vi "Version4.0.vi"() -> ()   [LabVIEW 2012]
uses:
  <vilib>/Instr/_visa.llb/VISA Configure Serial Port (Instr).vi
  Function_Set/Debug/Function_Set.dll
panel:
  in  "选项卡控件":T1(tab)
  in  "查询 2":bool
  in  "Other:":string
  in  "Save This Shot":bool
  out "Shots:":i32
  in  "Save This Notes":bool
  in  "Other Notes:":string
  out "Shot's situation:":string
  out "Shots:":i32
  out "Notes:":string
  in  "查询":bool
  in  "Options":u16(ring) caption="Choose File:" items=["2014-5-27梁一寒-Notes.txt", "2014-5-27梁一寒.txt", "2014-5-27袁鹏-Notes.txt", "2014-5-27袁鹏.txt", "20140527_110114.txt", "20140527_110114combined.txt", "20140527_110235.txt", "20140527_110235combined.txt"]
  in  "Initial Folder Path:":path
  in  "透镜位置：":dbl
  in  "靶位置：":dbl
  in  "激光能量：":dbl
  in  "实验员":u16(ring)
  in  "查找实验员":u16(ring)
  in  "搜索结果":u16(ring) caption="查找结果:" items=["2014-5-27梁一寒-Notes.txt", "2014-5-27梁一寒.txt"]
  in  "?":bool
  in  "Your Own:":u16(ring) items=["2, 0, 3, 2"]
  in  "FrameStartTriggerMode":T2(ring)
  in  "AcquisitionMode":T3(ring)
  in  "ExposureMode":T4(ring)
  in  "AVT SDK Demon":bool
  out "CCD ID":string
  out "ExposureMode":string
  out "ExposureValue":u32
  out "AcquisitionMode":string
  out "FrameStartTriggerMode":string
  in  "ExposureValue":u32
  in  "CameraStart":bool
  in  "CameraStop":bool
  in  "CameraSet":bool
  in  "CameraGet":bool
  in  "CameraSetAll":bool
  in  "path to JPEG file":path caption="Path of the Pic"
  out "new picture":picture caption="Pic"
  in  "OPEN":bool
  in  "端口选择":refnum<visa-resource-name>="COM1"
  in  "baud rate":u32=9600
  in  "data bits":u16=8
  in  "stop bits":u16(ring)=10 items=["1.0"=10, "1.5"=15, "2.0"=20]
  in  "flow control":u16(ring) items=["None"=0, "XON/XOFF"=1, "RTS/CTS"=2, "DTR/DSR"=4]
  in  "timeout":u32=10
  in  "RS485地址":string="12"
  in  "读取间隔(s)":dbl=1.0 caption="Delay Time (s)"
  in  "数据文件夹":string="data"
  in  "记录说明":string="test"
  out "数据路径":path
  in  "parity (0:none)":enum16{"None", "Odd", "Even", "Mark", "Space"}(ring)
  in  "记录所有读取数据?":bool
  out "已记录数据点":u32 caption="recorded number"
  in  "stop":bool
  out "电离规图表":dbl(graph)
  out "电阻规图表":dbl(graph)
  out "已读取数据点":i32
  out "预定耗时":dbl
  out "实际耗时":dbl
  in  "临界压强(Pa)":dbl=8.0
  in  "圈数":i32
  in  "X边长（mm）":dbl
  in  "VISA resource name":refnum<visa-resource-name>="COM1"
  in  "确认":bool
  in  "X轴速度mm/s":dbl(knob) scale=0.0..100.0
  in  "Y边长（mm）":dbl
  in  "Y轴速度mm/s":dbl(knob) scale=0.0..100.0
  out "进度条":dbl(slide) scale=0.0..100.0
  in  "设置速度":bool
  in  "baud rate 2":u32=9600
  in  "VISA resource name 2":refnum<visa-resource-name>="COM1"
  in  "data bits 2":u16=8 min=5 max=8 step=1
  in  "parity":u16(ring) items=["None", "Odd", "Even", "Mark", "Space"]
  in  "stop bits 2":u16(ring)=10 items=["1.0"=10, "1.5"=15, "2.0"=20]
  in  "timeout (ms)":u32=10000
  in  "flow control 2":u16(ring) items=["None"=0, "XON/XOFF"=1, "RTS/CTS"=2, "DTR/DSR"=4]
  in  "Input\nbuffer size":u32=4096
  in  "激光器端口设置完毕":bool
  in  "读取激光器字符串":string
  in  "控制器端口设置完毕":bool
  in  "baud rate 3":u32=9600
  in  "VISA resource name 3":refnum<visa-resource-name>="COM1"
  in  "data bits 3":u16=8 min=5 max=8 step=1
  in  "parity 2":u16(ring) items=["None", "Odd", "Even", "Mark", "Space"]
  in  "stop bits 3":u16(ring)=10 items=["1.0"=10, "1.5"=15, "2.0"=20]
  in  "timeout (ms) 2":u32=10000
  in  "flow control 3":u16(ring) items=["None"=0, "XON/XOFF"=1, "RTS/CTS"=2, "DTR/DSR"=4]
  in  "Input buffer size 2":u32=4096
  in  "字符串输出":bool
  in  "直接使用字符串输入：":string
  in  "启动总开关":bool
  in  "All the commands":path
  in  "选项卡控件 2":enum32{"单轴控制", "四轴控制", "同步控制"}(tab)
  in  "单轴输入":bool
  in  "Number of Pulses":i16
  in  "模式转换":bool
  in  "回到机械原点":bool
  in  "选择轴":u16(ring)=1 items=["轴1"=1, "轴2"=2, "轴3"=3, "轴4"=4]
  in  "轴 4":i16
  in  "轴 5":i16
  in  "轴 6":i16
  in  "轴1 2":i16
  in  "模式转换 2":bool
  in  "多轴输入":bool
  in  "模式转换 3":bool
  in  "轴1":i16
  in  "轴2":i16
  in  "轴3":i16
  in  "轴4":i16
  in  "同步运作":bool
  out "正在移动":bool
  in  "询问状态":bool
  in  "Parameter":string
  in  "轴":u16(ring)=1 items=["未定义", "轴1", "轴2", "轴3", "轴4"]
  out "情况":string
  in  "速度设置":bool
  in  "加速时间（ms）":i32
  in  "最大速度（PPS）":i32
  in  "最小速度（PPS）":i32
  in  "轴 3":u16(ring)=1 items=["未定义", "轴1", "轴2", "轴3", "轴4"]
  in  "返回位置":bool
  out "位置返回值":string
  in  "步长设置":bool
  in  "轴 2":u16(ring)=1 items=["未定义", "轴1", "轴2", "轴3", "轴4"]
  in  "分割步长":u16(ring) items=["0.36°;1000p/c;1μm"=2, "0.18°;2000p/c;0.5μm"=4, "0.036°;10000p/c;0.1μm"=20, "0.018°;20000p/c;0.05μm"=40, "0.0036°;100000p/c;0.01μm"=200]
  in  "全部减速停止":bool
  in  "轴4减速停止":bool
  in  "轴3减速停止":bool
  in  "轴2减速停止":bool
  in  "轴1减速停止":bool
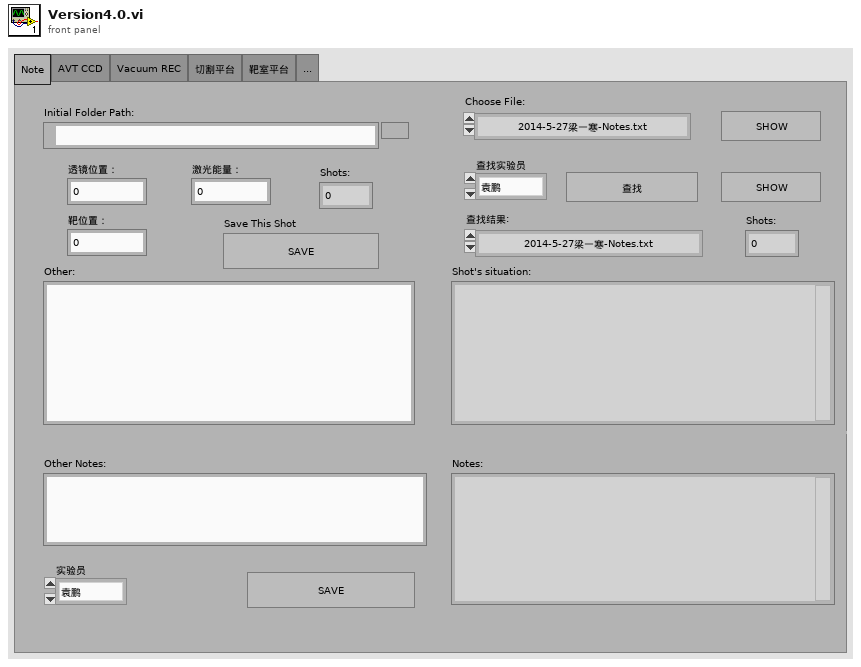
[diagram p1: front panel]
types:
  T1 = enum32{"Note", "AVT CCD", "Vacuum REC", "切割平台", "靶室平台", "..."}
  T2 = enum16{"默认", "Freerun", "SyncIn1", "SyncIn2", "FixedRate", "Software"}
  T3 = enum16{"默认", "Continuous", "SingleFrame", "MultiFrame", "Recorder"}
  T4 = enum16{"默认", "Manual", "Auto", "AutoOnce", "External"}
  T5 = enum16{"open", "replace", "create", "open or create", "replace or create", "replace or create with confirmation"}
  T6 = typedef "imagedata.ctl" = cluster{"image type":i32, "image depth":i32, "image":u8[], "mask":u8[], "colors":u32[], "Rectangle":cluster{"left":i16, "top":i16, "right":i16, "bottom":i16}}
  T7 = cluster{"Resister":dbl, "Ionization":dbl, "time":string, "Ionization":dbl, "Ionization":dbl, u32, i32}
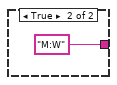
[diagram p4: hidden frame]
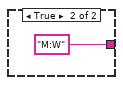
[diagram p11: hidden frame]
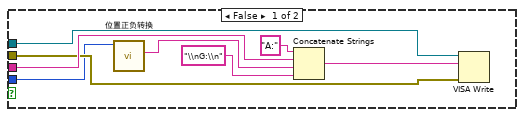
[diagram p13: hidden frame]
diagram:
  n1 = while {
    tunnel: "选项卡控件" -> [w19]
    stop <- w20 continue-if-true
    n2 = property on="Options" class="Ring (严格)"() -> ("Strings []"=w15:string[])  [unwired: 2 in, 2 out]
    n3 = property on="查找实验员" class="Ring (严格)"() -> ("RingText.Text"=w16:string)  [unwired: 2 in, 2 out]
    n4 = property on="实验员" class="Ring (严格)"() -> ("RingText.Text"=w17:string)  [unwired: 2 in, 2 out]
    n5 = property on="搜索结果" class="Ring (严格)"() -> ("RingText.Text"=w4:string)  [unwired: 2 in, 2 out]
    n6 = Array Size(array=w15) -> (size(s)=w14:i32)
    n7 = Equal?(x=T1."Note", y=w19) -> (x = y?=w20:bool)
    n8 = Not Equal?(x="查询", y="查询 2") -> (x != y?=w3:bool)
    n9 = Equal?(x="查询", y=w3) -> (x = y?=w8:bool)
    n10 = case shown="真" "Save This Shot" {
      tunnel: "Initial Folder Path:" -> [_ w97]
      tunnel: w17 -> [_ w85]
      frame False {
      }
      frame True {
        n11 = property on="Shots:" class="DigNum (严格)"() -> ("Value"=w93:i32)  [unwired: 2 in, 2 out]
        n12 = Decrement(x=w93) -> (x-1=w92:i32)
        n13 = Get Date/Time String(date format (0)=enum16{"short", "long", "abbreviated"}."short" ("日期格式(0)")) -> (date string=w108:string)  [unwired: 2 in, 1 out]
        n14 = feedback #1(1.0 ("x")) -> (w100:dbl)
        n15 = Increment(x=w100) -> (x+1=w98:dbl)
        "Shots:" <- w98
        n16 = feedback-in #1(w98) -> ()
        n17 = Search and Replace String(replace all?=TRUE ("替换全部？(F)"), input string=w108, search string="/" ("搜索字符串"), replace string="-" ("替换字符串(\"\")")) -> (result string=w105:string)  [unwired: 4 in, 3 out]
        n18 = Concatenate Strings(w105, "-" ("字符串"), w85, ".txt" ("字符串")) -> (w109:string)
        n19 = Build Path(base path=w97, name or relative path=w109) -> (appended path=w110:path)
        n20 = Open/Create/Replace File(file path (use dialog)=w110, operation (0:open)=T5."open or create" ("操作(0:open)"), access (0:read/write)=enum16{"read/write", "read-only", "write-only"}."read/write" ("权限(0:read/write)")) -> (refnum out=w102:refnum<file>)  [unwired: 3 in, 2 out]
        n21 = Number To Decimal String(number=w92) -> (decimal integer string=w96:string)  [unwired: 1 in]
        n22 = Concatenate Strings("NO." ("字符串"), w96, ": ;透镜位置: %f ;靶位置: %f ;激光能量: %f ;Other: %s\\n" ("格式字符串")) -> (w90:string)
        n23 = Set File Position(refnum=w102, from (0:start)=enum16{"start", "end", "current"}."end" ("自（0:起始）")) -> (refnum out=w101:refnum<file>)  [unwired: 2 in, 1 out]
        n24 = Format Into String(format string=w90, initial string=w101, "透镜位置：", "靶位置：", "激光能量：", "Other:") -> ()  [unwired: 1 in, 2 out]
      }
    }
    n25 = List Folder(path="Initial Folder Path:") -> (path out=w7:path, filenames=w11:string[])  [unwired: 3 in, 2 out]
    n26 = case shown="真" "Save This Notes" {
      tunnel: "Initial Folder Path:" -> [_ w68]
      tunnel: w17 -> [_ w66]
      frame False {
      }
      frame True {
        n27 = Get Date/Time String(date format (0)=enum16{"short", "long", "abbreviated"}."short" ("日期格式(0)")) -> (date string=w79:string)  [unwired: 2 in, 1 out]
        n28 = Search and Replace String(replace all?=TRUE ("替换全部？(F)"), input string=w79, search string="/" ("搜索字符串"), replace string="-" ("替换字符串(\"\")")) -> (result string=w70:string)  [unwired: 4 in, 3 out]
        n29 = Concatenate Strings(w70, "-" ("字符串"), w66, "-Notes.txt" ("字符串")) -> (w69:string)
        n30 = Build Path(base path=w68, name or relative path=w69) -> (appended path=w80:path)
        n31 = Open/Create/Replace File(file path (use dialog)=w80, operation (0:open)=T5."open or create" ("操作(0:open)"), access (0:read/write)=enum16{"read/write", "read-only", "write-only"}."read/write" ("权限(0:read/write)")) -> (refnum out=w73:refnum<file>)  [unwired: 3 in, 2 out]
        n32 = Set File Position(refnum=w73, from (0:start)=enum16{"start", "end", "current"}."end" ("自（0:起始）")) -> (refnum out=w72:refnum<file>)  [unwired: 2 in, 1 out]
        n33 = Format Into String(format string="Other Notes: %s\\n\\n" ("格式字符串"), initial string=w72, "Other Notes:") -> ()  [unwired: 1 in, 2 out]
      }
    }
    n34 = case shown="真" "?" {
      tunnel: w16 -> [_ w31]
      tunnel: w15 -> [_ w30]
      tunnel: w14 -> [_ w29]
      frame False {
      }
      frame True {
        n35 = while {
          tunnel: w30 -> [w38]
          tunnel: w31 -> [w37]
          tunnel: w29 -> [w36]
          i -> [w34]
          stop <- w35 stop-if-true
          n36 = Equal?(x=w36, y=w34) -> (x = y?=w35:bool)
          n37 = Decrement(x=w34) -> (x-1=w33:i32)
          n38 = Index Array(array=w38, index=w33) -> (element=w32:string)
          n39 = Search and Replace String(input string=w32, search string=w37) -> (number of replacements=w39:i32)  [unwired: 6 in, 3 out]
          n40 = Not Equal To 0?(x=w39) -> (x != 0?=w40:bool)
          n41 = case shown="真" w40 {
            tunnel: w32 -> [_ w43]
            frame False {
            }
            frame True {
              n42 = feedback #2() -> (w42:string[])  [unwired: 1 in]
              n43 = Build Array (concatenate)(w42, w43) -> (w41:string[])
              n44 = feedback-in #2(w41) -> ()
              n45 = property on="搜索结果" class="Ring (严格)"("Strings []"=w41) -> ()  [unwired: 2 in, 2 out]
            }
          }
        }
      }
    }
    n46 = property on="Options" class="Ring (严格)"("Strings []"=w11) -> ()  [unwired: 2 in, 2 out]
    n47 = Index Array(array=w11, index="Options") -> (element=w6:string)
    n48 = case shown="真" w8 {
      tunnel: w7 -> [w25 w28]
      tunnel: w6 -> [_ w27]
      tunnel: [w23 w26] -> w5
      tunnel: w4 -> [w24 _]
      frame False {
        n49 = Build Path(base path=w25, name or relative path=w24) -> (appended path=w23:path)
      }
      frame True {
        n50 = Build Path(base path=w28, name or relative path=w27) -> (appended path=w26:path)
      }
    }
    n51 = case shown="真" w3 {
      tunnel: w5 -> [_ w45]
      frame False {
      }
      frame True {
        n52 = Path To String(path=w45) -> (string=w44:string)
        n53 = call "时间延迟2"() -> ()  [unwired: 11 in, 1 out]
        n54 = Search and Replace String(input string=w44, search string="Notes" ("搜索字符串")) -> (number of replacements=w47:i32)  [unwired: 6 in, 3 out]
        n55 = Not Equal To 0?(x=w47) -> (x != 0?=w46:bool)
        n56 = case shown="真" w46 {
          tunnel: w45 -> [w49 w63]
          frame False {
            n57 = Open/Create/Replace File(file path (use dialog)=w49, operation (0:open)=T5."open" ("操作(0:open)"), access (0:read/write)=enum16{"read/write", "read-only", "write-only"}."read-only" ("权限(0:read/write)")) -> (refnum out=w60:refnum<file>)  [unwired: 3 in, 2 out]
            n58 = Read from Text File(file (use dialog)=w60) -> (text=w56:string)  [unwired: 3 in, 3 out]
            n59 = Search and Replace String(replace all?=TRUE ("替换全部？(F)"), input string=w56, search string="\n" ("搜索字符串"), replace string="\n\n" ("替换字符串(\"\")")) -> (result string=w53:string, number of replacements=→"Shots:":i32)  [unwired: 4 in, 2 out]
            n60 = Search and Replace String(replace all?=TRUE ("替换全部？(F)"), input string=w53, search string=";" ("搜索字符串"), replace string="\n" ("替换字符串(\"\")")) -> (result string=→"Shot's situation:":string)  [unwired: 4 in, 3 out]
          }
          frame True {
            n61 = Read from Text File(file (use dialog)=w63) -> (text=→"Notes:":string)  [unwired: 3 in, 3 out]
          }
        }
      }
    }
    n62 = call "时间延迟"() -> ()  [unwired: 11 in, 1 out]
  }
  n63 = while {
    tunnel: "选项卡控件" -> [w117]
    stop <- w118 continue-if-true
    n64 = case shown="真" "OPEN" {
      frame False {
      }
      frame True {
        n65 = call <vilib>:"Read JPEG File.vi"("path to JPEG file"="path to JPEG file") -> ("image data"=w128:T6)  [unwired: 8 in, 2 out]
        n66 = call <vilib>:"Draw Flattened Pixmap.vi"("image data"=w128) -> ("new picture"=→"new picture":picture)  [unwired: 8 in]
      }
    }
    n67 = case shown="真" "CameraStart" {
      frame False {
      }
      frame True {
        n68 = dll-call lib="F:/Kun's Test/Function_Set/Debug/Function_Set.dll" fn="CameraStart"() -> ()  [unwired: 4 in, 2 out]
      }
    }
    n69 = case shown="真" "CameraStop" {
      frame False {
      }
      frame True {
        n70 = dll-call lib="F:/Kun's Test/Function_Set/Debug/Function_Set.dll" fn="CameraStop"() -> ()  [unwired: 4 in, 2 out]
      }
    }
    n71 = case shown="真" "CameraSetAll" {
      frame False {
      }
      frame True {
        n72 = property on="Your Own:" class="Ring (严格)"() -> ("RingText.Text"=w131:string)  [unwired: 2 in, 2 out]
        n73 = Scan From String(format string="%d, %d, %d, %d" ("格式字符串"), input string=w131) -> (output 1=w133:i32, output 2=w134:i32, output 3=w135:i32, output 4=w136:i32)  [unwired: 6 in, 3 out]
        n74 = dll-call lib="F:/Kun's Test/Function_Set/Debug/Function_Set.dll" fn="CameraModeSet"("EM"=w133, "EV"=w134, "AM"=w135, "FSTM"=w136) -> ()  [unwired: 8 in, 2 out]
      }
    }
    n75 = case shown="真" "CameraGet" {
      frame False {
      }
      frame True {
        n76 = dll-call lib="F:/Kun's Test/Function_Set/Debug/Function_Set.dll" fn="CameraModeGet"("ExposureMode"="Manual", "ExposureValue"=u32 0, "AcquisitionMode"="Continuous", "FrameStartTriggerMode"="Freerun") -> ("ExposureMode"=→"ExposureMode":string, "ExposureValue"=→"ExposureValue":u32, "AcquisitionMode"=→"AcquisitionMode":string, "FrameStartTriggerMode"=→"FrameStartTriggerMode":string)  [unwired: 4 in, 2 out]
      }
    }
    n77 = Equal?(x=T1."AVT CCD", y=w117) -> (x = y?=w118:bool)
    n78 = case shown="真" "AVT SDK Demon" {
      frame False {
      }
      frame True {
        n79 = call <vilib>:"System Exec.vi"("working directory"=path "D:/Allied Vision Technologies/GigESDK/bin-pc", "command line"="cmd /cSampleViewer.exe") -> ()  [unwired: 6 in, 4 out]
      }
    }
    n80 = case shown="真" "CameraSet" {
      tunnel: "ExposureValue" -> [_ w156]
      tunnel: "ExposureMode" -> [_ w155]
      tunnel: "AcquisitionMode" -> [_ w154]
      tunnel: "FrameStartTriggerMode" -> [_ w153]
      frame False {
      }
      frame True {
        n81 = dll-call lib="F:/Kun's Test/Function_Set/Debug/Function_Set.dll" fn="CameraModeSet"("EM"=w155, "EV"=w156, "AM"=w154, "FSTM"=w153) -> ("返回类型"=→"CCD ID":string)  [unwired: 7 in, 2 out]
      }
    }
    n82 = case shown="真" "CameraSetAll" {
      tunnel: "ExposureMode" -> [_ w140]
      tunnel: "ExposureValue" -> [_ w139]
      tunnel: "AcquisitionMode" -> [_ w138]
      tunnel: "FrameStartTriggerMode" -> [_ w137]
      frame False {
      }
      frame True {
        n83 = Format Into String(format string="%d, %d, %d, %d" ("格式字符串"), w140, w139, w138, w137) -> (resulting string=w143:string)  [unwired: 2 in, 1 out]
        n84 = feedback #3() -> (w142:string[])  [unwired: 1 in]
        n85 = Build Array (concatenate)(w142, w143) -> (w141:string[])
        n86 = feedback-in #3(w141) -> ()
        n87 = property on="Your Own:" class="Ring (严格)"("Strings []"=w141) -> ()  [unwired: 2 in, 2 out]
      }
    }
  }
  n88 = while {
    tunnel: "选项卡控件" -> [w162]
    stop <- w161 continue-if-true
    w212 = FALSE  # Enable Termination Char (T)
    # "要记得给移位寄存器一个适当的初始值，虽然本程序中电阻电离移位寄存器无初始值不会带来错误。"
    n89 = Current VI's Path() -> (path=w204:path)
    n90 = Equal?(x=T1."Vacuum REC", y=w162) -> (x = y?=w161:bool)
    n91 = call "newfilewithexp.vi"("路径"=w204, "数据文件夹"="数据文件夹", "记录说明"="记录说明", "读取间隔(s)"="读取间隔(s)") -> ("数据路径"=→"数据路径":path, "refnum out for 4column"=w183:refnum<file>, "refnum out for 3column"=w181:refnum<file>, "error out"=w180:errorcluster)  [unwired: 1 in, 7 out]
    n92 = call-poly "VISA Configure Serial Port"("VISA resource name"="端口选择", "timeout (10sec)"="timeout", "Enable Termination\nChar (T)"=w212, "baud rate (9600)"="baud rate", "data bits (8)"="data bits", "parity (0:none)"="parity (0:none)", "stop bits (10: 1 bit)"="stop bits", "flow control (0:none)"="flow control") -> ("VISA resource name out"=w209:refnum<visa-resource-name>, "error out"=w184:errorcluster)  [unwired: 1 in, 5 out]
    n93 = Merge Errors(w180, w184) -> (w192:errorcluster)
    n94 = flat-sequence {
      tunnel: "RS485地址" -> [w232]
      tunnel: "读取间隔(s)" -> [w233]
      tunnel: "记录所有读取数据?" -> [w234]
      tunnel: w192 -> [w235]
      tunnel: w209 -> [w236]
      tunnel: [w236] -> w229
      tunnel: [w235] -> w228
      tunnel: [w234] -> w227
      tunnel: [w233] -> w226
      tunnel: [w232] -> w225
      tunnel: [w231] -> w224
      tunnel: "临界压强(Pa)" -> [w230]
      tunnel: [w230] -> w223
      tunnel: [w258] -> w222
      tunnel: [w237] -> w221
      tunnel: w229 -> [w260]
      tunnel: w228 -> [w259]
      tunnel: w227 -> [w256]
      tunnel: w226 -> [w255]
      tunnel: w225 -> [w254]
      tunnel: [w253] -> w220
      tunnel: w224 -> [w253]
      tunnel: [w252] -> w219
      tunnel: [w251] -> w218
      tunnel: w223 -> [w250]
      tunnel: [w249] -> w217
      tunnel: [w243] -> w216
      tunnel: [w238] -> w215
      tunnel: [w297] -> w207
      tunnel: [w298] -> w208
      tunnel: w222 -> [w298]
      tunnel: w221 -> [w297]
      tunnel: w220 -> [w295]
      tunnel: w219 -> [w289]
      tunnel: w218 -> [w292]
      tunnel: w217 -> [w290]
      tunnel: w216 -> [w291]
      tunnel: [w291] -> w197
      tunnel: [w290] -> w176
      tunnel: [w289] -> w175
      tunnel: [w288] -> w178
      tunnel: [w287] -> w177
      tunnel: w215 -> [w286]
      tunnel: [w286] -> w191
      frame #0 {
        n95 = Tick Count (ms)() -> (millisecond timer value=w231:u32)
      }
      frame #1 {
        w248 = 0.0 ("Ionization")
        n96 = Initialize Array(0.0 ("element"), 1 ("dimension size"), 4 ("dimension size")) -> (w246:dbl[][])
        n97 = Initialize Array(0.0 ("element"), 1 ("dimension size"), 3 ("dimension size")) -> (w239:dbl[][])
        n98 = while {
          tunnel: w260 -> [w285]
          tunnel: w259 -> [w284]
          tunnel: w254 -> [w281]
          tunnel: [w267] -> w258
          tunnel: [w282] -> w237
          shift-right: [w268] -> w249
          shift-left: u32 0 -> [w278]
          shift-right: [w262] -> _
          shift-left: w248 -> [w277]
          tunnel: w255 -> [w283]
          tunnel: w256 -> [w274]
          tunnel: [w261] -> w252
          tunnel: [w283] -> w251
          shift-right: [w263] -> _
          shift-left: w248 -> [w276]
          tunnel: w250 -> [w273]
          shift-right: [w271] -> w243
          shift-left: w246 -> [w272]
          shift-right: [w269] -> w238
          shift-left: w239 -> [w270]
          i -> [w279]
          stop <- w264 stop-if-true
          # "4col raw data array"
          # "3col combined array"
          n99 = call "Time Delay"("Delay Time (s)"=w283) -> ()  [unwired: 1 in, 10 out]
          n100 = call "GetPressure.vi"("Address of RS485"=w281, "error in (no error)"=w284, "VISA resource name"=w285) -> ("error out"=w267:errorcluster, "Ionization"=w262:dbl, "Resister"=w263:dbl, "VISA resource name out"=w282:refnum<visa-resource-name>, "time"=w280:string)  [unwired: 1 in, 3 out]
          "电阻规图表" <- w263
          "电离规图表" <- w262
          n101 = Increment(x=w279) -> (x+1=w261:i32)
          "已读取数据点" <- w261
          n102 = Unbundle By Name(w267) -> ("status"=w265:bool)
          n103 = Bundle("Resister"=w263, "Ionization"=w262, "time"=w280, "Ionization"=w276, "Ionization"=w277, w278, w279) -> (w275:T7)  [unwired: 1 out]
          n104 = call "2D_data_array.vi"("input cluster"=w275, "input 4column array"=w272, "input combined 3column array"=w270, "critical pressure"=w273, "record all data points?"=w274) -> ("output 4column array"=w271:dbl[][], "output combined 3column array"=w269:dbl[][], "recorded number out"=w268:u32)  [unwired: 4 out]
          "已记录数据点" <- w268
          n105 = Or(x="stop", y=w265) -> (x .or. y?=w264:bool)
        }
      }
      frame #2 {
        n106 = Multiply(x=w292, y=w289) -> (x*y=w288:dbl)
        "预定耗时" <- w288
        n107 = Tick Count (ms)() -> (millisecond timer value=w296:u32)
        n108 = Subtract(x=w296, y=w295) -> (x-y=w294:u32)
        n109 = Divide(x=w294, y=1000.0) -> (x/y=w287:dbl)
        "实际耗时" <- w287
      }
    }
    n110 = VISA Close(VISA resource name=w207, error in (no error)=w208) -> (error out=w170:errorcluster)
    n111 = Delete From Array(array=w197, index (row)=0) -> (array with subset deleted=w198:dbl[][])  [unwired: 2 in, 1 out]
    n112 = Delete From Array(array=w191, index (row)=0) -> (array with subset deleted=w188:dbl[][])  [unwired: 2 in, 1 out]
    n113 = call "data_combination.vi"("input combined data array"=w188) -> ("recorded combined data number"=w174:i32, "output combined data array"=w185:dbl[][])  [unwired: 9 out]
    n114 = Array To Spreadsheet String(array=w198, 3:"%#f" ("format string")) -> (spreadsheet string=w182:string)  [unwired: 1 out]
    n115 = Array To Spreadsheet String(array=w185, 3:"%#f" ("format string")) -> (spreadsheet string=w179:string)  [unwired: 1 out]
    n116 = Write to Text File(file (use dialog)=w183, text=w182, error in=w180) -> (refnum out=w194:refnum<file>, error out=w193:errorcluster)  [unwired: 2 out]
    n117 = call "endstr.vi"("实际耗时"=w177, "预定耗时"=w178, "error in"=w193, "已读取数据点"=w175, "已记录数据点"=w176, "refnum in"=w194) -> ("error out"=w196:errorcluster, "refnum out"=w195:refnum<file>)  [unwired: 4 out]
    n118 = Write to Text File(file (use dialog)=w181, text=w179, error in=w180) -> (refnum out=w173:refnum<file>, error out=w172:errorcluster)  [unwired: 2 out]
    n119 = call "endstr.vi"("实际耗时"=w177, "预定耗时"=w178, "error in"=w172, "已读取数据点"=w175, "已记录数据点"=w174, "refnum in"=w173) -> ("error out"=w186:errorcluster, "refnum out"=w187:refnum<file>)  [unwired: 4 out]
    n120 = Close File(refnum=w195, error in=w196) -> (error out=w168:errorcluster)  [unwired: 1 out]
    n121 = Close File(refnum=w187, error in=w186) -> (error out=w169:errorcluster)  [unwired: 1 out]
    n122 = Merge Errors(w168, w169, w170) -> (w171:errorcluster)
    n123 = call <vilib>:"Simple Error Handler.vi"("error in (no error)"=w171) -> ()  [unwired: 1 in, 8 out]
  }
  n124 = while {
    tunnel: "选项卡控件" -> [w301]
    stop <- w300 continue-if-true
    w352 = u16 16  # I/O Receive Buffer mask
    w367 = u16 16  # I/O Receive Buffer mask
    n125 = Equal?(x=w301, y=T1."靶室平台") -> (x = y?=w300:bool)
    n126 = call-poly "VISA Configure Serial Port"("VISA resource name"="VISA resource name 2", "timeout (10sec)"="timeout (ms)", "termination char\n(0xA = '\\n' = LF)"=u8 10 ("termination char\n(0xA = '\\n' = LF)"), "Enable Termination\nChar (T)"=TRUE ("End read on termination character?"), "baud rate (9600)"="baud rate 2", "data bits (8)"="data bits 2", "parity (0:none)"="parity", "stop bits (10: 1 bit)"="stop bits 2", "flow control (0:none)"="flow control 2") -> ("VISA resource name out"=w366:refnum<visa-resource-name>, "error out"=w364:errorcluster)  [unwired: 1 in, 4 out]
    n127 = call-poly "VISA Configure Serial Port"("VISA resource name"="VISA resource name 3", "timeout (10sec)"="timeout (ms) 2", "termination char\n(0xA = '\\n' = LF)"=u8 10 ("termination char\n(0xA = '\\n' = LF)"), "Enable Termination\nChar (T)"=TRUE ("End read on termination character?"), "baud rate (9600)"="baud rate 3", "data bits (8)"="data bits 3", "parity (0:none)"="parity 2", "stop bits (10: 1 bit)"="stop bits 3", "flow control (0:none)"="flow control 3") -> ("VISA resource name out"=w351:refnum<visa-resource-name>, "error out"=w349:errorcluster)  [unwired: 1 in, 4 out]
    n128 = Open/Create/Replace File(file path (use dialog)="All the commands") -> (refnum out=w345:refnum<file>)  [unwired: 1 in, 6 out]
    n129 = VISA Set I/O Buffer Size(VISA resource name=w366, mask (16)=w367, size (4096)="Input\nbuffer size", error in (no error)=w364) -> (VISA resource name out=w363:refnum<visa-resource-name>, error out=w362:errorcluster)
    n130 = VISA Set I/O Buffer Size(VISA resource name=w351, mask (16)=w352, size (4096)="Input buffer size 2", error in (no error)=w349) -> (VISA resource name out=w348:refnum<visa-resource-name>, error out=w344:errorcluster)
    n131 = while {
      tunnel: w363 -> [w430]
      tunnel: w362 -> [w433]
      tunnel: w348 -> [w431]
      tunnel: [w416] -> w346
      tunnel: w345 -> [w415]
      tunnel: w344 -> [w414]
      tunnel: [w413] -> w342
      tunnel: [w412] -> w340
      tunnel: [w411] -> w338
      tunnel: [w410] -> w337
      tunnel: [w409] -> w336
      tunnel: [w408] -> w335
      tunnel: [w407] -> w333
      tunnel: [w406] -> w331
      tunnel: [w405] -> w330
      tunnel: [w404] -> w328
      tunnel: [w403] -> w327
      tunnel: [w402] -> w325
      tunnel: [w401] -> w324
      tunnel: [w400] -> w322
      tunnel: [w399] -> w321
      tunnel: [w398] -> w319
      tunnel: [w397] -> w318
      tunnel: [w396] -> w316
      tunnel: [w395] -> w315
      tunnel: [w394] -> w314
      tunnel: [w393] -> w312
      tunnel: [w392] -> w311
      tunnel: [w387] -> w309
      tunnel: [w386] -> w308
      tunnel: [w380] -> w305
      tunnel: [w379] -> w304
      tunnel: [w378] -> w303
      tunnel: [w377] -> w302
      stop <- "启动总开关" continue-if-true
      n132 = case shown="真" "控制器端口设置完毕" {
        tunnel: w430 -> [_ w536]
        tunnel: w433 -> [_ w534]
        tunnel: [_ w523] -> w428
        tunnel: [_ w497] -> w427
        tunnel: [_ w522] -> w426
        tunnel: [_ w521] -> w425
        tunnel: [_ w520] -> w424
        tunnel: [_ w519] -> w423
        tunnel: [_ w518] -> w422
        tunnel: [_ w517] -> w421
        tunnel: [_ w516] -> w413
        tunnel: [_ w515] -> w412
        tunnel: [_ w514] -> w411
        tunnel: [_ w513] -> w410
        tunnel: [_ w512] -> w409
        tunnel: [_ w511] -> w408
        tunnel: [_ w498] -> w407
        tunnel: [_ w510] -> w406
        tunnel: [_ w509] -> w405
        tunnel: [_ w508] -> w404
        tunnel: [_ w507] -> w403
        tunnel: [_ w496] -> w402
        tunnel: [_ w506] -> w401
        tunnel: [_ w505] -> w400
        tunnel: [_ w504] -> w399
        tunnel: [_ w503] -> w398
        tunnel: [_ w502] -> w397
        tunnel: [_ w499] -> w394
        tunnel: [_ w494] -> w393
        tunnel: [_ w493] -> w392
        tunnel: [_ w491] -> w390
        tunnel: [_ w490] -> w388
        tunnel: [_ w489] -> w387
        tunnel: [_ w488] -> w386
        tunnel: [_ w483] -> w384
        tunnel: [_ w482] -> w382
        tunnel: [_ w481] -> w381
        tunnel: [_ w480] -> w380
        tunnel: [_ w479] -> w379
        tunnel: [_ w478] -> w378
        tunnel: [_ w477] -> w377
        frame False {
        }
        frame True {
          n133 = Number To Decimal String(number="选择轴") -> (decimal integer string=w531:string)  [unwired: 1 out]
          n134 = VISA Write(VISA resource name=w536, write buffer="M:W+P3+P3+P3+P3\\nG:\\nR:W\\n" ("写入缓冲区"), error in (no error)=w534) -> (VISA resource name out=w486:refnum<visa-resource-name>, error out=w485:errorcluster)  [unwired: 1 out]
          n135 = case shown="真" "全部减速停止" {
            tunnel: w486 -> [_ w666]
            tunnel: [_ w665] -> w517
            tunnel: w485 -> [_ w664]
            tunnel: [_ w663] -> w516
            tunnel: [_ w662] -> w511
            frame False {
            }
            frame True {
              w665 = "L:W\\n" ("写入缓冲区")
              n136 = VISA Write(VISA resource name=w666, write buffer=w665, error in (no error)=w664) -> (VISA resource name out=w662:refnum<visa-resource-name>, error out=w663:errorcluster)  [unwired: 1 out]
            }
          }
          n137 = case shown="真" "轴1减速停止" {
            tunnel: w486 -> [_ w686]
            tunnel: [_ w685] -> w521
            tunnel: w485 -> [_ w684]
            tunnel: [_ w683] -> w505
            tunnel: [_ w682] -> w504
            frame False {
            }
            frame True {
              w685 = "L:1\\n" ("写入缓冲区")
              n138 = VISA Write(VISA resource name=w686, write buffer=w685, error in (no error)=w684) -> (VISA resource name out=w682:refnum<visa-resource-name>, error out=w683:errorcluster)  [unwired: 1 out]
            }
          }
          n139 = case shown="真" "轴3减速停止" {
            tunnel: w486 -> [_ w676]
            tunnel: [_ w675] -> w519
            tunnel: w485 -> [_ w674]
            tunnel: [_ w673] -> w514
            tunnel: [_ w672] -> w513
            frame False {
            }
            frame True {
              w675 = "L:3\\n" ("写入缓冲区")
              n140 = VISA Write(VISA resource name=w676, write buffer=w675, error in (no error)=w674) -> (VISA resource name out=w672:refnum<visa-resource-name>, error out=w673:errorcluster)  [unwired: 1 out]
            }
          }
          n141 = case shown="真" "轴2减速停止" {
            tunnel: w486 -> [_ w681]
            tunnel: [_ w680] -> w520
            tunnel: w485 -> [_ w679]
            tunnel: [_ w678] -> w510
            tunnel: [_ w677] -> w509
            frame False {
            }
            frame True {
              w680 = "L:2\\n" ("写入缓冲区")
              n142 = VISA Write(VISA resource name=w681, write buffer=w680, error in (no error)=w679) -> (VISA resource name out=w677:refnum<visa-resource-name>, error out=w678:errorcluster)  [unwired: 1 out]
            }
          }
          n143 = case shown="真" "轴4减速停止" {
            tunnel: w486 -> [_ w671]
            tunnel: [_ w670] -> w518
            tunnel: w485 -> [_ w669]
            tunnel: [_ w668] -> w515
            tunnel: [_ w667] -> w512
            frame False {
            }
            frame True {
              w670 = "L:4\\n" ("写入缓冲区")
              n144 = VISA Write(VISA resource name=w671, write buffer=w670, error in (no error)=w669) -> (VISA resource name out=w667:refnum<visa-resource-name>, error out=w668:errorcluster)  [unwired: 1 out]
            }
          }
          n145 = case shown="真" "回到机械原点" {
            tunnel: w531 -> [_ w693]
            tunnel: w486 -> [_ w690]
            tunnel: w485 -> [_ w689]
            tunnel: [_ w688] -> w503
            tunnel: [_ w687] -> w502
            frame False {
            }
            frame True {
              n146 = Concatenate Strings("H:" ("字符串"), w693, "\\n" ("字符串")) -> (w691:string)
              n147 = VISA Write(VISA resource name=w690, write buffer=w691, error in (no error)=w689) -> (VISA resource name out=w687:refnum<visa-resource-name>, error out=w688:errorcluster)  [unwired: 1 out]
            }
          }
          n148 = case shown="真" "字符串输出" {
            tunnel: w486 -> [_ w661]
            tunnel: [_ "直接使用字符串输入："] -> w522
            tunnel: w485 -> [_ w659]
            tunnel: [_ w658] -> w508
            tunnel: [_ w657] -> w507
            frame False {
            }
            frame True {
              n149 = VISA Write(VISA resource name=w661, write buffer="直接使用字符串输入：", error in (no error)=w659) -> (VISA resource name out=w657:refnum<visa-resource-name>, error out=w658:errorcluster)  [unwired: 1 out]
            }
          }
          n150 = case shown="真" "单轴输入" {
            tunnel: w531 -> [_ w637]
            tunnel: "Number of Pulses" -> [_ w636]
            tunnel: w486 -> [_ w631]
            tunnel: [_ w635] -> w523
            tunnel: w485 -> [_ w634]
            tunnel: [_ w633] -> w506
            tunnel: [_ w632] -> w496
            frame False {
            }
            frame True {
              n151 = case shown="真" "模式转换" {
                tunnel: w637 -> [w642 w655]
                tunnel: w631 -> [w641 w652]
                tunnel: w634 -> [w640 w651]
                tunnel: w636 -> [w639 w650]
                tunnel: [_ w649] -> w635
                tunnel: [_ w648] -> w632
                tunnel: [_ w647] -> w633
                frame False {
                  n152 = call "位置正负转换.vi"("x"=w639) -> ("连接的字符串 2"=w645:string)  [unwired: 10 out]
                  n153 = Concatenate Strings("A:" ("字符串"), w642, w645, "\\nG:\\n" ("字符串")) -> (w643:string)
                  n154 = VISA Write(VISA resource name=w641, write buffer=w643, error in (no error)=w640) -> ()  [unwired: 3 out]
                }
                frame True {
                  n155 = call "位置正负转换.vi"("x"=w650) -> ("连接的字符串 2"=w654:string)  [unwired: 10 out]
                  n156 = Concatenate Strings("M:" ("字符串"), w655, w654, "\\nG:\\n" ("字符串")) -> (w649:string)
                  n157 = VISA Write(VISA resource name=w652, write buffer=w649, error in (no error)=w651) -> (VISA resource name out=w648:refnum<visa-resource-name>, error out=w647:errorcluster)  [unwired: 1 out]
                }
              }
            }
          }
          n158 = case shown="真" "多轴输入" {
            tunnel: [_ w617] -> w499
            tunnel: w486 -> [_ w616]
            tunnel: [_ w615] -> w498
            tunnel: w485 -> [_ w614]
            tunnel: [_ w613] -> w497
            frame False {
            }
            frame True {
              n159 = call "位置正负转换.vi"("x"="轴1 2") -> ("连接的字符串 2"=w622:string)  [unwired: 10 out]
              n160 = call "位置正负转换.vi"("x"="轴 6") -> ("连接的字符串 2"=w621:string)  [unwired: 10 out]
              n161 = call "位置正负转换.vi"("x"="轴 5") -> ("连接的字符串 2"=w620:string)  [unwired: 10 out]
              n162 = call "位置正负转换.vi"("x"="轴 4") -> ("连接的字符串 2"=w619:string)  [unwired: 10 out]
              n163 = case shown="假" "模式转换 2" {
                tunnel: ["A:W" ("字符串") "M:W" ("字符串")] -> w627
                frame False {
                }
                frame True {
                }
              }
              n164 = Concatenate Strings(w627, w622, w621, w620, w619, "\\nG:\\n" ("字符串")) -> (w613:string)
              n165 = VISA Write(VISA resource name=w616, write buffer=w613, error in (no error)=w614) -> (VISA resource name out=w617:refnum<visa-resource-name>, error out=w615:errorcluster)  [unwired: 1 out]
            }
          }
          n166 = for {
            N: 1 -> [_]
            tunnel: [w543] -> w479
            tunnel: [w542] -> w480
            tunnel: w486 -> [w540]
            tunnel: w485 -> [w539]
            tunnel: [w538] -> w482
            tunnel: [w537] -> w481
            n167 = case shown="真" "询问状态" {
              tunnel: [_ w556] -> w543
              tunnel: [_ w555] -> w542
              tunnel: w540 -> [_ w551]
              tunnel: w539 -> [_ w550]
              tunnel: [_ w545] -> w538
              tunnel: [_ w544] -> w537
              frame False {
              }
              frame True {
                n168 = Number To Decimal String(number="轴") -> (decimal integer string=w547:string)  [unwired: 1 out]
                n169 = Concatenate Strings("?:" ("字符串"), "Parameter", w547) -> (w545:string)
                n170 = VISA Write(VISA resource name=w551, write buffer=w545, error in (no error)=w550) -> (VISA resource name out=w554:refnum<visa-resource-name>, error out=w553:errorcluster)  [unwired: 1 out]
                n171 = VISA Read(VISA resource name=w554, byte count=u32 20 ("字节总数"), error in (no error)=w553) -> (VISA resource name out=w555:refnum<visa-resource-name>, read buffer=w544:string, error out=w556:errorcluster)  [unwired: 1 out]
                "情况" <- w544
              }
            }
          }
          n172 = for {
            N: 1 -> [_]
            tunnel: [w577] -> w488
            tunnel: [w576] -> w489
            tunnel: w486 -> [w574]
            tunnel: w485 -> [w573]
            tunnel: [w572] -> w490
            n173 = case shown="真" "步长设置" {
              tunnel: [_ w588] -> w577
              tunnel: [_ w587] -> w576
              tunnel: w574 -> [_ w580]
              tunnel: w573 -> [_ w579]
              tunnel: [_ w578] -> w572
              frame False {
              }
              frame True {
                n174 = Number To Decimal String(number="轴 2") -> (decimal integer string=w584:string)  [unwired: 1 out]
                n175 = Number To Decimal String(number="分割步长") -> (decimal integer string=w582:string)  [unwired: 1 out]
                n176 = Concatenate Strings("S:" ("字符串"), w584, w582, "\\n" ("字符串")) -> (w578:string)
                n177 = VISA Write(VISA resource name=w580, write buffer=w578, error in (no error)=w579) -> (VISA resource name out=w587:refnum<visa-resource-name>, error out=w588:errorcluster)  [unwired: 1 out]
              }
            }
          }
          n178 = for {
            N: 1 -> [_]
            tunnel: w486 -> [w594]
            tunnel: [w593] -> w494
            tunnel: [w592] -> w493
            tunnel: w485 -> [w591]
            tunnel: [w589] -> w491
            n179 = case shown="真" "速度设置" {
              tunnel: w594 -> [_ w600]
              tunnel: [_ w599] -> w593
              tunnel: [_ w598] -> w592
              tunnel: w591 -> [_ w597]
              tunnel: [_ w595] -> w589
              frame False {
              }
              frame True {
                n180 = Number To Decimal String(number="轴 3") -> (decimal integer string=w610:string)  [unwired: 1 out]
                n181 = Number To Decimal String(number="最小速度（PPS）") -> (decimal integer string=w608:string)  [unwired: 1 out]
                n182 = Number To Decimal String(number="最大速度（PPS）") -> (decimal integer string=w605:string)  [unwired: 1 out]
                n183 = Number To Decimal String(number="加速时间（ms）") -> (decimal integer string=w602:string)  [unwired: 1 out]
                n184 = Concatenate Strings("D:" ("字符串"), w610, "S" ("字符串"), w608, "F" ("字符串"), w605, "R" ("字符串"), w602, "\\n" ("字符串")) -> (w595:string)
                n185 = VISA Write(VISA resource name=w600, write buffer=w595, error in (no error)=w597) -> (VISA resource name out=w598:refnum<visa-resource-name>, error out=w599:errorcluster)  [unwired: 1 out]
              }
            }
          }
          n186 = for {
            N: 1 -> [_]
            tunnel: [w562] -> w477
            tunnel: [w561] -> w478
            tunnel: w486 -> [w559]
            tunnel: w485 -> [w558]
            tunnel: [w557] -> w483
            n187 = case shown="真" "返回位置" {
              tunnel: [_ w571] -> w562
              tunnel: [_ w570] -> w561
              tunnel: w559 -> [_ w568]
              tunnel: w558 -> [_ w566]
              tunnel: [_ w563] -> w557
              frame False {
              }
              frame True {
                n188 = VISA Write(VISA resource name=w568, write buffer="Q:\\n" ("写入缓冲区"), error in (no error)=w566) -> (VISA resource name out=w569:refnum<visa-resource-name>, error out=w567:errorcluster)  [unwired: 1 out]
                n189 = VISA Read(VISA resource name=w569, byte count=u32 50 ("字节总数"), error in (no error)=w567) -> (VISA resource name out=w570:refnum<visa-resource-name>, read buffer=w563:string, error out=w571:errorcluster)  [unwired: 1 out]
                "位置返回值" <- w563
              }
            }
          }
        }
      }
      n190 = case shown="真" "激光器端口设置完毕" {
        tunnel: w431 -> [_ w441]
        tunnel: w430 -> [_ w440]
        tunnel: [_ w439] -> w418
        tunnel: w414 -> [_ w438]
        tunnel: [_ w437] -> w396
        tunnel: [_ w436] -> w395
        frame False {
        }
        frame True {
          n191 = while {
            tunnel: w441 -> [w456]
            tunnel: w440 -> [w450]
            tunnel: [w446] -> w439
            tunnel: w438 -> [w445]
            tunnel: [w443] -> w437
            tunnel: [w442] -> w436
            stop <- "同步运作" continue-if-true
            n192 = VISA Read(VISA resource name=w456, byte count=u32 20 ("字节总数")) -> (VISA resource name out=w448:refnum<visa-resource-name>, read buffer=w455:string)  [unwired: 1 in, 2 out]
            n193 = String Length(string="读取激光器字符串") -> (length=w452:i32)
            n194 = Scan From String(format string="读取激光器字符串", input string=w455, error in=w445) -> (offset past scan=w453:u32, error out=w444:errorcluster)  [unwired: 1 in, 3 out]
            n195 = Equal?(x=w452, y=w453) -> (x = y?=w451:bool)
            n196 = case shown="真" w451 {
              selector: w451 -> [_ w461]
              tunnel: w450 -> [_ w463]
              tunnel: w448 -> [_ w462]
              tunnel: [_ w460] -> w446
              tunnel: w444 -> [_ w459]
              tunnel: [_ w458] -> w443
              tunnel: [_ w457] -> w442
              frame False {
              }
              frame True {
                n197 = VISA Clear(VISA resource name=w462) -> ()  [unwired: 1 in, 2 out]
                n198 = call "位置正负转换.vi"("x"="轴1") -> ("连接的字符串 2"=w469:string)  [unwired: 10 out]
                n199 = call "位置正负转换.vi"("x"="轴2") -> ("连接的字符串 2"=w468:string)  [unwired: 10 out]
                n200 = call "位置正负转换.vi"("x"="轴3") -> ("连接的字符串 2"=w467:string)  [unwired: 10 out]
                n201 = call "位置正负转换.vi"("x"="轴4") -> ("连接的字符串 2"=w464:string)  [unwired: 10 out]
                n202 = case shown="假" "模式转换 3" {
                  tunnel: ["A:W" ("字符串") "M:W" ("字符串")] -> w473
                  frame False {
                  }
                  frame True {
                  }
                }
                n203 = call "时间延迟3"() -> ()  [unwired: 2 in, 10 out]
                n204 = Concatenate Strings(w473, w469, w468, w467, w464, "\\nG:\\n" ("字符串")) -> (w460:string)
                n205 = VISA Write(VISA resource name=w463, write buffer=w460, error in (no error)=w459) -> (VISA resource name out=w458:refnum<visa-resource-name>, error out=w457:errorcluster)  [unwired: 1 out]
                "正在移动" <- w461
              }
            }
          }
        }
      }
      n206 = Concatenate Strings("单独控制：" ("字符串"), w428, "四轴控制：" ("字符串"), w427, w426, w425, w424, w423, w422, w421, "同步控制：" ("字符串"), w418, "速度设置：" ("字符串"), w390, "步长设置：" ("字符串"), w388, "询问位置：" ("字符串"), w384, "询问情况：" ("字符串"), w382, w381) -> (w417:string)
      n207 = Write to Text File(file (use dialog)=w415, text=w417) -> (refnum out=w416:refnum<file>)  [unwired: 1 in, 3 out]
    }
    n208 = Close File(refnum=w346) -> ()  [unwired: 1 in, 2 out]
    n209 = VISA Close(VISA resource name=w325, error in (no error)=w324) -> (error out=w326:errorcluster)
    n210 = VISA Close(VISA resource name=w314, error in (no error)=w333) -> (error out=w334:errorcluster)
    n211 = VISA Close(VISA resource name=w305, error in (no error)=w304) -> (error out=w307:errorcluster)
    n212 = VISA Close(VISA resource name=w309, error in (no error)=w308) -> (error out=w310:errorcluster)
    n213 = VISA Close(VISA resource name=w311, error in (no error)=w312) -> (error out=w313:errorcluster)
    n214 = VISA Close(VISA resource name=w303, error in (no error)=w302) -> (error out=w306:errorcluster)
    n215 = VISA Close(VISA resource name=w335, error in (no error)=w342) -> (error out=w343:errorcluster)
    n216 = VISA Close(VISA resource name=w321, error in (no error)=w322) -> (error out=w323:errorcluster)
    n217 = VISA Close(VISA resource name=w337, error in (no error)=w338) -> (error out=w339:errorcluster)
    n218 = VISA Close(VISA resource name=w330, error in (no error)=w331) -> (error out=w332:errorcluster)
    n219 = VISA Close(VISA resource name=w336, error in (no error)=w340) -> (error out=w341:errorcluster)
    n220 = VISA Close(VISA resource name=w318, error in (no error)=w319) -> (error out=w320:errorcluster)
    n221 = VISA Close(VISA resource name=w327, error in (no error)=w328) -> (error out=w329:errorcluster)
    n222 = VISA Close(VISA resource name=w316, error in (no error)=w315) -> (error out=w317:errorcluster)
    n223 = call <vilib>:"Simple Error Handler.vi"("error in (no error)"=w326) -> ()  [unwired: 1 in, 8 out]
    n224 = call <vilib>:"Simple Error Handler.vi"("error in (no error)"=w334) -> ()  [unwired: 1 in, 8 out]
    n225 = call <vilib>:"Simple Error Handler.vi"("error in (no error)"=w307) -> ()  [unwired: 1 in, 8 out]
    n226 = call <vilib>:"Simple Error Handler.vi"("error in (no error)"=w310) -> ()  [unwired: 1 in, 8 out]
    n227 = call <vilib>:"Simple Error Handler.vi"("error in (no error)"=w313) -> ()  [unwired: 1 in, 8 out]
    n228 = call <vilib>:"Simple Error Handler.vi"("error in (no error)"=w306) -> ()  [unwired: 1 in, 8 out]
    n229 = call <vilib>:"Simple Error Handler.vi"("error in (no error)"=w343) -> ()  [unwired: 1 in, 8 out]
    n230 = call <vilib>:"Simple Error Handler.vi"("error in (no error)"=w323) -> ()  [unwired: 1 in, 8 out]
    n231 = call <vilib>:"Simple Error Handler.vi"("error in (no error)"=w339) -> ()  [unwired: 1 in, 8 out]
    n232 = call <vilib>:"Simple Error Handler.vi"("error in (no error)"=w332) -> ()  [unwired: 1 in, 8 out]
    n233 = call <vilib>:"Simple Error Handler.vi"("error in (no error)"=w341) -> ()  [unwired: 1 in, 8 out]
    n234 = call <vilib>:"Simple Error Handler.vi"("error in (no error)"=w320) -> ()  [unwired: 1 in, 8 out]
    n235 = call <vilib>:"Simple Error Handler.vi"("error in (no error)"=w329) -> ()  [unwired: 1 in, 8 out]
    n236 = call <vilib>:"Simple Error Handler.vi"("error in (no error)"=w317) -> ()  [unwired: 1 in, 8 out]
  }
  n237 = while {
    tunnel: "选项卡控件" -> [w697]
    stop <- w696 continue-if-true
    w698 = u16 0 items=["无", "XON/XOFF", "RTS/CTS", "XON/XOFF & RTS/CTS", "DTR/DSR", "XON/XOFF & DTR/DSR"] ("flow control (0:none)")
    w699 = u16 10 items=["1.0"=10, "1.5"=15, "2.0"=20] ("stop bits (10: 1 bit)")
    w709 = FALSE  # Enable Termination Char (T)
    w710 = u32 10000  # timeout (10sec)
    n238 = Equal?(x=w697, y=T1."靶室平台") -> (x = y?=w696:bool)
    n239 = call-poly "VISA Configure Serial Port"("VISA resource name"="VISA resource name", "timeout (10sec)"=w710, "Enable Termination\nChar (T)"=w709, "baud rate (9600)"=u32 19200, "data bits (8)"=u16 8, "parity (0:none)"=enum16{"None", "Odd", "Even", "Mark", "Space"}."None", "stop bits (10: 1 bit)"=w699, "flow control (0:none)"=w698) -> ("VISA resource name out"=w708:refnum<visa-resource-name>, "error out"=w707:errorcluster)  [unwired: 1 in, 5 out]
    n240 = for {
      N: "圈数" -> [w720]
      tunnel: w708 -> [w735]
      tunnel: w707 -> [w732]
      tunnel: [w722] -> w705
      tunnel: [w721] -> w704
      i -> [w715]
      n241 = flat-sequence {
        tunnel: w732 -> [w739]
        tunnel: w735 -> [w740]
        tunnel: [w738] -> w713
        tunnel: [w737] -> w712
        tunnel: [w768] -> w734
        tunnel: [w767] -> w733
        tunnel: [w766] -> w728
        tunnel: ["确认"] -> w723
        tunnel: w713 -> [w764]
        tunnel: w712 -> [w763]
        tunnel: w734 -> [w807]
        tunnel: w733 -> [w806]
        tunnel: [w805] -> w731
        tunnel: [w804] -> w730
        tunnel: [w803] -> w729
        tunnel: w728 -> [w803]
        tunnel: [w802] -> w724
        tunnel: w723 -> [w801]
        tunnel: w731 -> [w846]
        tunnel: w730 -> [w845]
        tunnel: w729 -> [w844]
        tunnel: [w843] -> w727
        tunnel: [w842] -> w726
        tunnel: [w841] -> w725
        tunnel: w724 -> [w841]
        tunnel: w727 -> [w881]
        tunnel: w726 -> [w880]
        tunnel: w725 -> [w879]
        tunnel: [w877] -> w722
        tunnel: [w876] -> w721
        frame #0 {
          n242 = case shown="真" FALSE {
            tunnel: w740 -> [w742 w756]
            tunnel: w739 -> [w741 w746]
            tunnel: [w742 w744] -> w738
            tunnel: [w741 w743] -> w737
            frame False {
            }
            frame True {
              n243 = Multiply ("乘")(x="Y轴速度mm/s", y=u16 800) -> (x*y=w752:u16)
              n244 = Multiply ("乘")(x="X轴速度mm/s", y=u16 800) -> (x*y=w760:u16)
              n245 = Number To Decimal String(number=w752) -> (decimal integer string=w751:string)  [unwired: 1 out]
              n246 = Number To Decimal String(number=w760) -> (decimal integer string=w759:string)  [unwired: 1 out]
              n247 = Concatenate Strings("VY," ("字符串"), w751, "\r" ("字符串")) -> (w748:string)
              n248 = Concatenate Strings("VX," ("字符串"), w759, "\r" ("字符串")) -> (w755:string)
              n249 = VISA Write(VISA resource name=w756, write buffer=w755, error in (no error)=w746) -> (VISA resource name out=w747:refnum<visa-resource-name>, error out=w745:errorcluster)  [unwired: 1 out]
              n250 = VISA Write(VISA resource name=w747, write buffer=w748, error in (no error)=w745) -> (VISA resource name out=w744:refnum<visa-resource-name>, error out=w743:errorcluster)  [unwired: 1 out]
            }
          }
        }
        frame #1 {
          n251 = case shown="真" "确认" {
            tunnel: [_ w800] -> w769
            tunnel: [_ w799] -> w770
            tunnel: [_ w793] -> w766
            tunnel: w764 -> [_ w791]
            tunnel: w763 -> [_ w790]
            frame False {
            }
            frame True {
              n252 = Multiply ("乘")(x="X边长（mm）", y=800.0) -> (x*y=w796:u16)
              n253 = Number To Decimal String(number=w796) -> (decimal integer string=w793:string)  [unwired: 1 out]
              n254 = Concatenate Strings("+X," ("字符串"), w793, "\r" ("字符串")) -> (w794:string)
              n255 = VISA Write(VISA resource name=w791, write buffer=w794, error in (no error)=w790) -> (VISA resource name out=w799:refnum<visa-resource-name>, error out=w800:errorcluster)  [unwired: 1 out]
            }
          }
          n256 = while {
            tunnel: w770 -> [w779]
            tunnel: w769 -> [w778]
            tunnel: [w773] -> w768
            tunnel: [w772] -> w767
            stop <- w771 stop-if-true
            n257 = property class="Instr"(reference=w779, error in=w778) -> (reference out=w780:refnum<visa-resource-name>, error out=w777:errorcluster, "Serial Settings:Number of Bytes at Serial Port"=w775:u32)
            n258 = Wait Until Next ms Multiple(millisecond multiple=u32 100 ("毫秒倍数")) -> ()  [unwired: 1 out]
            n259 = Not Equal To 0?(x=w775) -> (x != 0?=w774:bool)
            n260 = case shown="真" w774 {
              tunnel: w780 -> [_ w789]
              tunnel: w775 -> [_ w788]
              tunnel: w777 -> [_ w787]
              tunnel: [_ w786] -> w773
              tunnel: [_ w785] -> w772
              tunnel: [_ w781] -> w771
              frame False {
              }
              frame True {
                n261 = VISA Read(VISA resource name=w789, byte count=w788, error in (no error)=w787) -> (VISA resource name out=w786:refnum<visa-resource-name>, read buffer=w784:string, error out=w785:errorcluster)  [unwired: 1 out]
                n262 = String Length(string=w784) -> (length=w783:i32)
                n263 = Greater?(x=w783, y=3) -> (0:w781:bool)
              }
            }
          }
        }
        frame #2 {
          n264 = case shown="真" w801 {
            tunnel: [_ w820] -> w808
            tunnel: [_ w819] -> w809
            tunnel: w807 -> [_ w813]
            tunnel: w806 -> [_ w812]
            tunnel: [_ w811] -> w802
            frame False {
            }
            frame True {
              n265 = Multiply ("乘")(x="Y边长（mm）", y=800.0) -> (x*y=w816:u16)
              n266 = Number To Decimal String(number=w816) -> (decimal integer string=w811:string)  [unwired: 1 out]
              n267 = Concatenate Strings("+Y," ("字符串"), w811, "\r" ("字符串")) -> (w814:string)
              n268 = VISA Write(VISA resource name=w813, write buffer=w814, error in (no error)=w812) -> (VISA resource name out=w819:refnum<visa-resource-name>, error out=w820:errorcluster)  [unwired: 1 out]
            }
          }
          n269 = while {
            tunnel: [w825] -> w805
            tunnel: [w824] -> w804
            tunnel: w809 -> [w823]
            tunnel: w808 -> [w822]
            stop <- w821 stop-if-true
            n270 = property class="Instr"(reference=w823, error in=w822) -> (reference out=w830:refnum<visa-resource-name>, error out=w829:errorcluster, "Serial Settings:Number of Bytes at Serial Port"=w827:u32)
            n271 = Wait Until Next ms Multiple(millisecond multiple=u32 100 ("毫秒倍数")) -> ()  [unwired: 1 out]
            n272 = Not Equal To 0?(x=w827) -> (x != 0?=w826:bool)
            n273 = case shown="真" w826 {
              tunnel: w830 -> [_ w839]
              tunnel: w827 -> [_ w838]
              tunnel: w829 -> [_ w837]
              tunnel: [_ w836] -> w825
              tunnel: [_ w835] -> w824
              tunnel: [_ w831] -> w821
              frame False {
              }
              frame True {
                n274 = VISA Read(VISA resource name=w839, byte count=w838, error in (no error)=w837) -> (VISA resource name out=w836:refnum<visa-resource-name>, read buffer=w834:string, error out=w835:errorcluster)  [unwired: 1 out]
                n275 = String Length(string=w834) -> (length=w832:i32)
                n276 = Greater?(x=w832, y=3) -> (0:w831:bool)
              }
            }
          }
        }
        frame #3 {
          n277 = case shown="真" TRUE {
            tunnel: [_ w856] -> w847
            tunnel: [_ w855] -> w848
            tunnel: w846 -> [_ w851]
            tunnel: w845 -> [_ w850]
            tunnel: w844 -> [_ w849]
            frame False {
            }
            frame True {
              n278 = Concatenate Strings("-X," ("字符串"), w849, "\r" ("字符串")) -> (w852:string)
              n279 = VISA Write(VISA resource name=w851, write buffer=w852, error in (no error)=w850) -> (VISA resource name out=w855:refnum<visa-resource-name>, error out=w856:errorcluster)  [unwired: 1 out]
            }
          }
          n280 = while {
            tunnel: [w861] -> w843
            tunnel: [w860] -> w842
            tunnel: w848 -> [w859]
            tunnel: w847 -> [w858]
            stop <- w857 stop-if-true
            n281 = property class="Instr"(reference=w859, error in=w858) -> (reference out=w866:refnum<visa-resource-name>, error out=w865:errorcluster, "Serial Settings:Number of Bytes at Serial Port"=w863:u32)
            n282 = Wait Until Next ms Multiple(millisecond multiple=u32 100 ("毫秒倍数")) -> ()  [unwired: 1 out]
            n283 = Not Equal To 0?(x=w863) -> (x != 0?=w862:bool)
            n284 = case shown="真" w862 {
              tunnel: w866 -> [_ w875]
              tunnel: w863 -> [_ w874]
              tunnel: w865 -> [_ w873]
              tunnel: [_ w872] -> w861
              tunnel: [_ w871] -> w860
              tunnel: [_ w867] -> w857
              frame False {
              }
              frame True {
                n285 = VISA Read(VISA resource name=w875, byte count=w874, error in (no error)=w873) -> (VISA resource name out=w872:refnum<visa-resource-name>, read buffer=w870:string, error out=w871:errorcluster)  [unwired: 1 out]
                n286 = String Length(string=w870) -> (length=w868:i32)
                n287 = Greater?(x=w868, y=3) -> (0:w867:bool)
              }
            }
          }
        }
        frame #4 {
          n288 = case shown="真" TRUE {
            tunnel: [_ w891] -> w882
            tunnel: [_ w890] -> w883
            tunnel: w881 -> [_ w886]
            tunnel: w880 -> [_ w885]
            tunnel: w879 -> [_ w884]
            frame False {
            }
            frame True {
              n289 = Concatenate Strings("-Y," ("字符串"), w884, "\r" ("字符串")) -> (w887:string)
              n290 = VISA Write(VISA resource name=w886, write buffer=w887, error in (no error)=w885) -> (VISA resource name out=w890:refnum<visa-resource-name>, error out=w891:errorcluster)  [unwired: 1 out]
            }
          }
          n291 = while {
            tunnel: [w896] -> w877
            tunnel: [w895] -> w876
            tunnel: w883 -> [w894]
            tunnel: w882 -> [w893]
            stop <- w892 stop-if-true
            n292 = property class="Instr"(reference=w894, error in=w893) -> (reference out=w901:refnum<visa-resource-name>, error out=w900:errorcluster, "Serial Settings:Number of Bytes at Serial Port"=w898:u32)
            n293 = Wait Until Next ms Multiple(millisecond multiple=u32 100 ("毫秒倍数")) -> ()  [unwired: 1 out]
            n294 = Not Equal To 0?(x=w898) -> (x != 0?=w897:bool)
            n295 = case shown="真" w897 {
              tunnel: w901 -> [_ w910]
              tunnel: w898 -> [_ w909]
              tunnel: w900 -> [_ w908]
              tunnel: [_ w907] -> w896
              tunnel: [_ w906] -> w895
              tunnel: [_ w902] -> w892
              frame False {
              }
              frame True {
                n296 = VISA Read(VISA resource name=w910, byte count=w909, error in (no error)=w908) -> (VISA resource name out=w907:refnum<visa-resource-name>, read buffer=w905:string, error out=w906:errorcluster)  [unwired: 1 out]
                n297 = String Length(string=w905) -> (length=w903:i32)
                n298 = Greater?(x=w903, y=3) -> (0:w902:bool)
              }
            }
          }
        }
      }
      n299 = Add(x=1.0, y=w715) -> (x+y=w714:dbl)
      n300 = Divide(x=w714, y=w720) -> (x/y=w719:dbl)
      n301 = Multiply(x=w719, y=100.0) -> (x*y=→"进度条":dbl)
    }
    n302 = VISA Close(VISA resource name=w705, error in (no error)=w704) -> (error out=w706:errorcluster)
    n303 = call <vilib>:"Simple Error Handler.vi"("error in (no error)"=w706) -> ()  [unwired: 1 in, 8 out]
  }
